vi "Write Is Pure.vi"(8 "error in (no error)":errorcluster, 10 "Is Pure":bool, 11 "ZXing Options in":refnum<class "ZXing.lvclass">) -> (0 "error out":errorcluster, 3 "ZXing Options out":refnum<class "ZXing.lvclass">)   [LabVIEW 2020, in "feature_detection.lvlib" / "ZXing.lvclass"]
uses:
  ZXing.lvclass
  ZXing.lvclass/ZXing.ctl
  Field.ctl
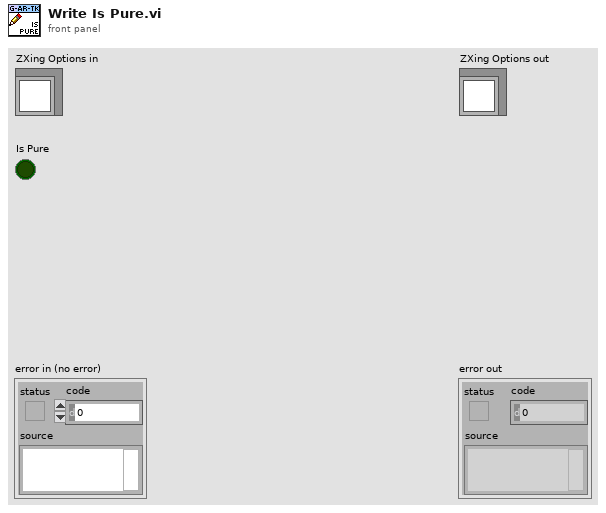
[diagram p1: front panel]
types:
  T1 = typedef "feature_detection.lvlib/ZXing.lvclass/Field.ctl" = enum8{"Try Harder", "Try Rotate", "Try Invert", "Try Downscale", "Is Pure", "Try Code 39 Ext Mode", "Return Errors", "Downscale Factor", "Min Line Count", "Max Number of Symbols", "Binarizer", "EAN Add On Symbol", "Text Mode", "Character Set", "Downscale Threshold"}
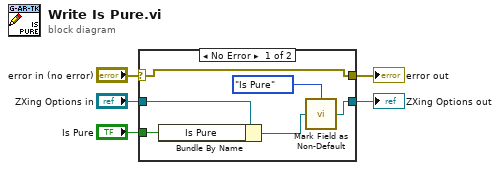
[diagram p0: block diagram]
diagram:
  n1 = case shown="No Error" "error in (no error)" {
    selector: "error in (no error)" -> [w11 w12]
    tunnel: [w11 w12] -> w4
    tunnel: [w7 w13] -> w2
    tunnel: "ZXing Options in" -> [w10 w13]
    tunnel: "Is Pure" -> [w8 _]
    frame No Error {
      n2 = Bundle By Name(cluster=w10, "Is Pure"=w8) -> (w9:refnum<class "ZXing.lvclass">)
      n3 = call "Mark Field as Non-Default.vi"("ZXing Options in"=w9, "Field"=Field."Is Pure") -> ("ZXing Options out"=w7:refnum<class "ZXing.lvclass">)
    }
    frame Error {
    }
  }
  "error out" <- w4
  "ZXing Options out" <- w2
